vi "Loader_BML.vi"(6 "Timeset between frms":u32=50, 7 "PinMap":path, 8 "error in (no error)":errorcluster, 9 "Pattern Name":string, 10 "BML Frame Array":refnum<class "BML_Frame_Root.lvclass">[](array[class]), 11 "BML_DigiPattern_Generator.lvclass":refnum<class "DigiPattern_Generator.lvclass">) -> (0 "error out":errorcluster, 3 "BML_DigiPattern_Generator.lvclass out":refnum<class "DigiPattern_Generator.lvclass">)   [LabVIEW 2018, in "DigiPattern_Generator.lvclass"]
uses:
  DigiPattern_Generator.lvclass
  BML_Frame_Root/BML_Frame_Root.lvclass
  DigiPattern_Generator.lvclass/DigiPattern_Generator.ctl
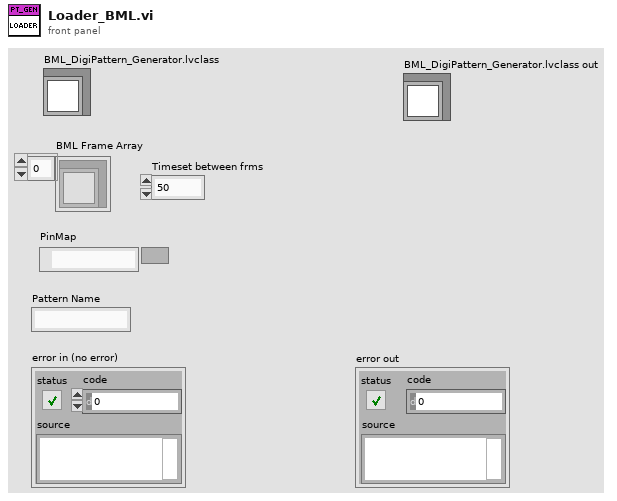
[diagram p1: front panel]
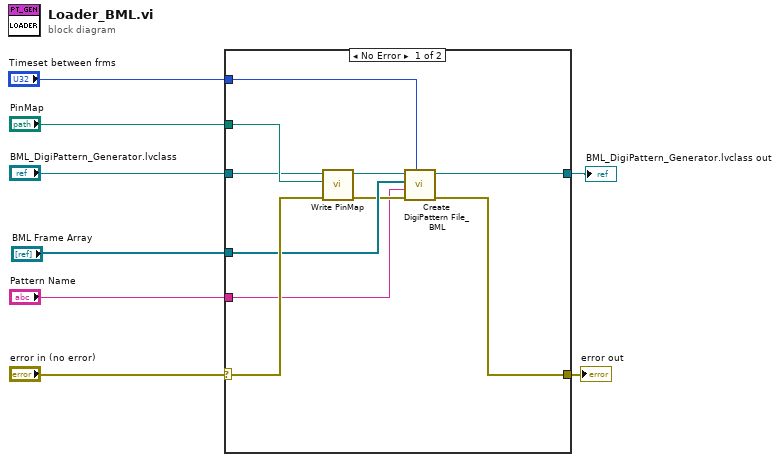
[diagram p0: block diagram]
diagram:
  n1 = case shown="No Error" "error in (no error)" {
    selector: "error in (no error)" -> [w15 w19]
    tunnel: "BML_DigiPattern_Generator.lvclass" -> [w17 w20]
    tunnel: "PinMap" -> [w18 _]
    tunnel: "BML Frame Array" -> [w14 _]
    tunnel: "Pattern Name" -> [w12 _]
    tunnel: [w11 w20] -> w4
    tunnel: [w10 w19] -> w3
    tunnel: "Timeset between frms" -> [w9 _]
    frame No Error {
      n2 = call "Write PinMap.vi"("error in (no error)"=w15, "PinMap"=w18, "BML_DigiPattern_Generator in"=w17) -> ("error out"=w13:errorcluster, "BML_DigiPattern_Generator out"=w16:refnum<class "DigiPattern_Generator.lvclass">)  [unwired: 7 in]
      n3 = call "Create DigiPattern File_BML.vi"("Timeset between frms"=w9, "error in (no error)"=w13, "Pattern Name"=w12, "BML Frame Array"=w14, "BML_DigiPattern_Generator.lvclass"=w16) -> ("error out"=w10:errorcluster, "BML_DigiPattern_Generator.lvclass out"=w11:refnum<class "DigiPattern_Generator.lvclass">)  [unwired: 5 in]
    }
    frame Error {
    }
  }
  "BML_DigiPattern_Generator.lvclass out" <- w4
  "error out" <- w3
